vi "Update Camera.vi"(11 "Main Controller Actor in":refnum<class "Main Controller Actor.lvclass">) -> (3 "Main Controller Actor out":refnum<class "Main Controller Actor.lvclass">)   [LabVIEW 2021, in "Main Controller Actor.lvclass"]
uses:
  Main Controller Actor.lvclass
  Main Controller Actor.lvclass/Main Controller Actor.ctl
  Globals.vi
  Camera/Camera.lvclass
  Element/Element.lvclass
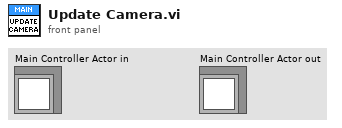
[diagram p1: front panel]
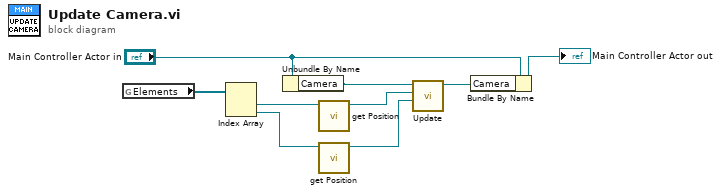
[diagram p0: block diagram]
diagram:
  n1 = global read "Globals.vi" "Elements"() -> (w8:refnum<class "Element.lvclass">[])
  n2 = Index Array(array=w8) -> (element #1=w5:refnum<class "Element.lvclass">, element #2=w3:refnum<class "Element.lvclass">)  [unwired: 2 in]
  n3 = Unbundle By Name("Main Controller Actor in") -> ("Camera"=w6:refnum<class "Camera.lvclass">)
  n4 = call "get Position.vi"("Element in"=w5) -> ("Position"=w4:refnum<class "Vector 2D.lvclass">)  [unwired: 10 in]
  n5 = call "get Position.vi"("Element in"=w3) -> ("Position"=w2:refnum<class "Vector 2D.lvclass">)  [unwired: 10 in]
  n6 = call "Update.vi"("Player 2 Position"=w2, "Player 1 Position"=w4, "Camera in"=w6) -> ("Camera out"=w1:refnum<class "Camera.lvclass">)  [unwired: 8 in]
  n7 = Bundle By Name(cluster="Main Controller Actor in", "Camera"=w1) -> (→"Main Controller Actor out":refnum<class "Main Controller Actor.lvclass">)
